vi "niFpgaXilinxIpExtension.vi"() -> ()   [LabVIEW 2020]
panel:
  in  "IP extension":string="lvxip"
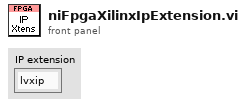
[diagram p1: front panel]
diagram:
